vi "backup_EnsTerm.vi"() -> ()   [LabVIEW 2019]
uses:
  <vilib>/Utility/error.llb/DialogType.ctl
  <vilib>/DAQmx/write.llb/DAQmx Write (Digital Bool 1Line 1Point).vi
  <vilib>/DAQmx/write.llb/DAQmx Write (Counter Frequency 1Chan 1Samp).vi
  <vilib>/DAQmx/miscellaneous.llb/DAQmx Fill In Error Info.vi
  <vilib>/DAQmx/create/channels.llb/DAQmx Create Channel (CO-Pulse Generation-Frequency).vi
  <vilib>/DAQmx/configure/timing.llb/DAQmx Timing (Implicit).vi
  <vilib>/addons/control/pid/pid.llb/PID (DBL).vi
  <vilib>/Utility/file.llb/Write Delimited Spreadsheet (string).vi
  <instrlib>/Agilent 34970/Agilent 34970.lvlib
  <resource>/objmgr/daqmx.rc
  <vilib>/addons/control/pid/NI_PID_pid.lvlib
  <instrlib>/Yokogawa WT200 Series/Yokogawa WT200 Series.lvlib
panel:
  out "temperature num cluster":T1
  out "Chart Temperatura":cluster{dbl, dbl, dbl, dbl, dbl, dbl}(graph)={21.505, 22.941, 24.092, 23.94, 23.972, 20.648}
  out "TP 2":dbl
  out "G. TP 2":cluster{dbl, "index":i32}(graph)
  out "TP 15":dbl
  out "TP 13":dbl
  out "TP 12":dbl
  out "TP 11":dbl
  out "TP 10":dbl
  out "TP 8":dbl
  out "TP 7":dbl
  out "TP 6":dbl
  out "TP 5":dbl
  out "TP 3":dbl
  out "TP 1":dbl
  out "G. TP 15":cluster{dbl, "index":i32}(graph)
  out "G. TP 13":cluster{dbl, "index":i32}(graph)
  out "G. TP 12":cluster{dbl, "index":i32}(graph)
  out "G. TP 11":cluster{dbl, "index":i32}(graph)
  out "G. TP 10":cluster{dbl, "index":i32}(graph)
  out "G. TP 8":cluster{dbl, "index":i32}(graph)
  out "G. TP 7":cluster{dbl, "index":i32}(graph)
  out "G. TP 6":cluster{dbl, "index":i32}(graph)
  out "G. TP 5":cluster{dbl, "index":i32}(graph)
  out "G. TP 3":cluster{dbl, "index":i32}(graph)
  out "G. TP 1":cluster{dbl, "index":i32}(graph)
  in  "Idenfier_Ens. Term.":string="medsETMA"
  in  "Idenfier_Freio":string="medsFreio"
  in  "Identifier_Watt":string="medsWatt"
  out "PL(E)":dbl
  out "PC(E)":dbl
  out "PC(T)":dbl
  out "PL(T)":dbl
  out "t":dbl
  out "Tensão de saída":dbl format="%.4f"
  out "Corrente de saída":dbl format="%.4f"
  out "watt num cluster":T2
  in  "Liga Fonte":bool
  out "Resposta":string
  out "Tradução":string
  in  "Parar motor":bool
  in  "Envia mensagem":bool
  in  "Enviar velocidade":bool
  in  "Seta carga":bool
  in  "Limite de tensão":dbl=30.0 min=0.0 max=30.0 step=0.5 format="%.4f"
  in  "Limite de corrente":dbl=0.075 min=0.0 max=0.4 step=0.01 format="%.4f"
  in  "Mensagem":T3(ring)=enum."Read power"
  in  "Velocidade (RPM)":u16=1000 min=1000 max=10000 step=100
  in  "Parâmetros serial":T4={"Serial VCC"="COM7", "timeout"=2, "baud rate"=600, "flow control"=0, "data bits"=8, "parity"=enum."None", "stop bits"=10, "termination char"=FALSE} {"stop bits" items=["1.0"=10, "1.5"=15, "2.0"=20]; "flow control" items=["None", "XON/XOFF", "RTS/CTS", "XON/XOFF & RTS/CTS", "DTR/DSR", "XON/XOFF & DTR/DSR"]}
  in  "Medição contínua? WT230":bool=TRUE
  in  "Realiza medição WT230":bool=TRUE
  out "Chart potencia numeric":T5(graph)={"PC(A)"=0.0, "PC(B)"=7.200000254670158e-05, "PC(T)"=7.200000254670158e-05, "PL(A)"=0.0, "PL(B)"=0.0, "PL(T)"=0.0, "PC(E)"=1.0970638990402222, "PL(E)"=1.0099999904632568}
  out "Chart corrente numeric":cluster{"I(A)":dbl, "I(B)":dbl, "I(E)":dbl}(graph)={"I(A)"=0.0, "I(B)"=0.0, "I(E)"=0.14239999651908875}
  out "Chart tensão numeric":cluster{"V(A)":dbl, "V(B)":dbl, "V(E)":dbl}(graph)={"V(A)"=0.0, "V(B)"=0.0, "V(E)"=228.25999450683594}
  in  "Tempo de integração (s)":u32=5 min=1 max=60 step=1
  in  "SP:":dbl(slide)=25.0 min=0.0 max=0.0 scale=25.0..70.0
  out "MV":dbl(graph)
  in  "Ts":dbl=1.0
  out "PV":dbl
  out "Process variable and Setpoint":cluster{"initial PV":dbl, "SP:":dbl}(graph)
  in  "PID gains":T6={"proportional gain (Kc)"=39.6, "integral time (Ti, min)"=14.617, "derivative time (Td, min)"=0.0} {"derivative time (Td, min)" format="%.3f"; "integral time (Ti, min)" format="%.3f"; "proportional gain (Kc)" format="%.6f"}
  in  "Frequency":dbl=1.0 format="%.6f"
  out "Duty Cycle":sgl=0.1 min=0.1 max=99.9 format="%#_6f"
  in  "Forno_on":bool=TRUE
  out "Iteration":i32
  in  "STOP":bool
  out "Temperature CH4 [degC]":dbl
  out "Temperature CH9 [degC]":dbl
  out "Time":dbl=300.0 format="%<%H:%M:%S>t"
  in  "Idenfier_Forno":string="medsForno"
  # "Temperaturas do Motor/Freio"
  # "Temperaturas dos Termopares"
  # "Gráficos:"
  # "Nome do arquivo:"
  # "Legenda:"
  # "TP 1: Termopar do Capacitor C011"
  # "TP 8: Termopar do CI SMPS IC100"
  # "TP 2: Termopar do Capacitor C009"
  # "TP 10: Termopar do Indutor L100"
  # "TP 3: Termopar do Choke L001"
  # "TP 11: Termopar do Capacitor C112"
  # "TP 5: Termopar do Capacitor C006"
  # "TP 12: Termopar do Capacitor C504"
  # "TP 6: Termopar do Fusível F002"
  # "TP 13: Termopar do Microcontrolador IC601"
  # "TP 7: Termopar do Conector CN204"
  # "TP 15: Termopar do Dissipador"
  # "Freio"
  # "Wattímetro WT230 Yokogawa"
  # "Controle de Temperatura do Forno"
  # "Controles"
  # "Geral"
  # "Respostas do Sistema em Malha Fechada"
  # "Controles"
  # "Medidas"
  # "Respostas temporais"
  # "Medidas"
  # "Controles"
  # "Inversor de Frequência"
  # "Comandos"
  # "Medidas"
  # "Parâmetros Serial"
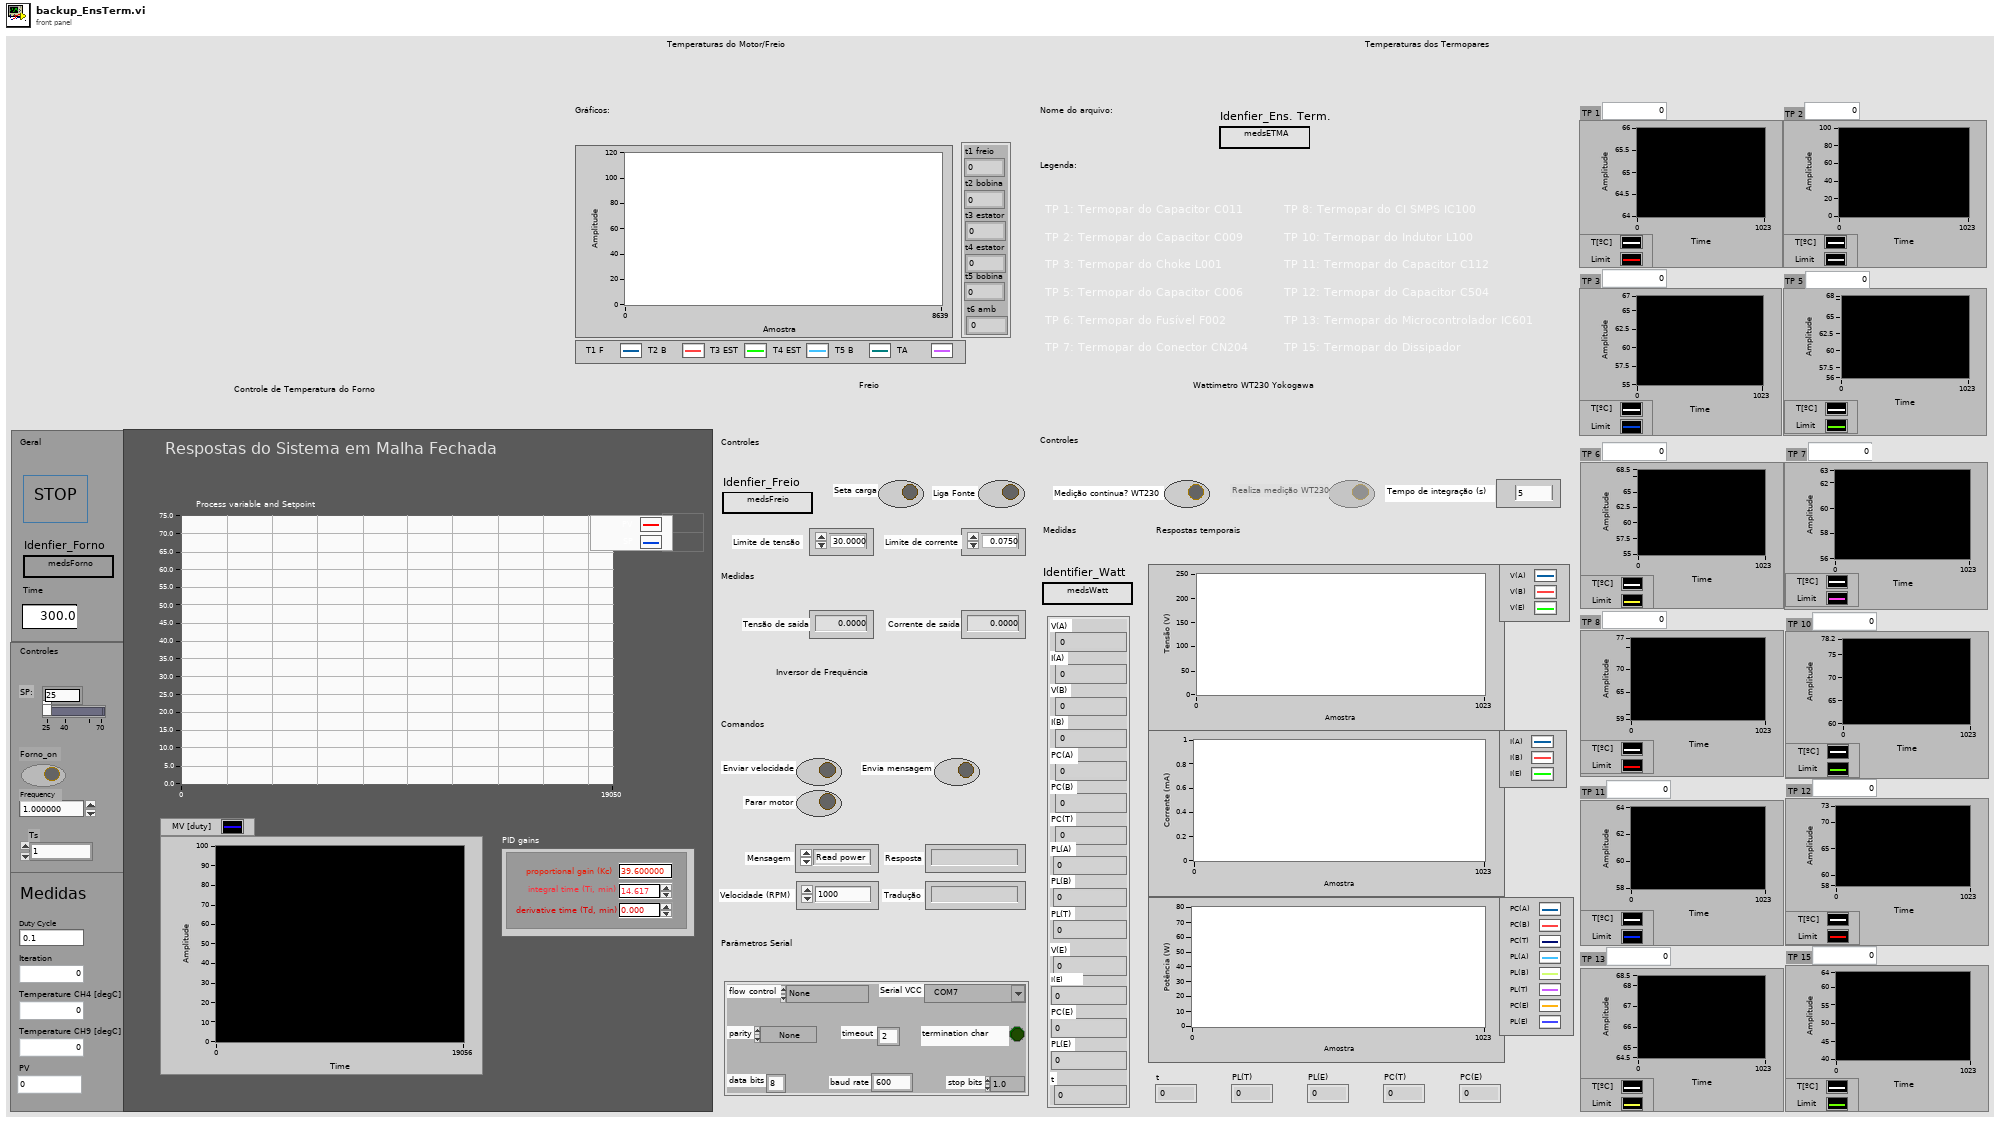
[diagram p1: front panel]
types:
  T1 = cluster{"t1 freio":dbl, "t2 bobina":dbl, "t5 bobina":dbl, "t4 estator":dbl, "t3 estator":dbl, "t6 amb":dbl}
  T2 = cluster{"V(A)":dbl, "I(A)":dbl, "V(B)":dbl, "I(B)":dbl, "PC(A)":dbl, "PC(B)":dbl, "PC(T)":dbl, "PL(T)":dbl, "PL(B)":dbl, "PL(A)":dbl, "V(E)":dbl, "PL(E)":dbl, "PC(E)":dbl, "I(E)":dbl, "t":dbl}
  T3 = enum16{"Read set speed", "Read operation status", "Read power", "Read starting trials", "Read bus voltage", "Read temperature", "Read power limitation", "Read PWM mode", "Read PWM frequency", "Read real speed"}
  T4 = cluster{"Serial VCC":refnum<visa-resource-name>, "timeout":u32, "baud rate":u32, "flow control":u16, "data bits":u16, "parity":enum16{"None", "Odd", "Even", "Mark", "Space"}, "stop bits":u16, "termination char":bool}
  T5 = cluster{"PC(A)":dbl, "PC(B)":dbl, "PC(T)":dbl, "PL(A)":dbl, "PL(B)":dbl, "PL(T)":dbl, "PC(E)":dbl, "PL(E)":dbl}
  T6 = cluster{"proportional gain (Kc)":dbl, "integral time (Ti, min)":dbl, "derivative time (Td, min)":dbl}
  T7 = enum16{"Start Comm.", "End Comm.", "Wait", "Send Static Message", "Set Speed"}
  T8 = enum16{"Thermocouple", "Thermistor", "RTD", "4-Wire RTD", "Default (Last)"}
  T9 = enum8{"Enabled", "Disabled", "Disabled and Grayed Out"}
  T10 = typedef "DialogType.ctl" = u16
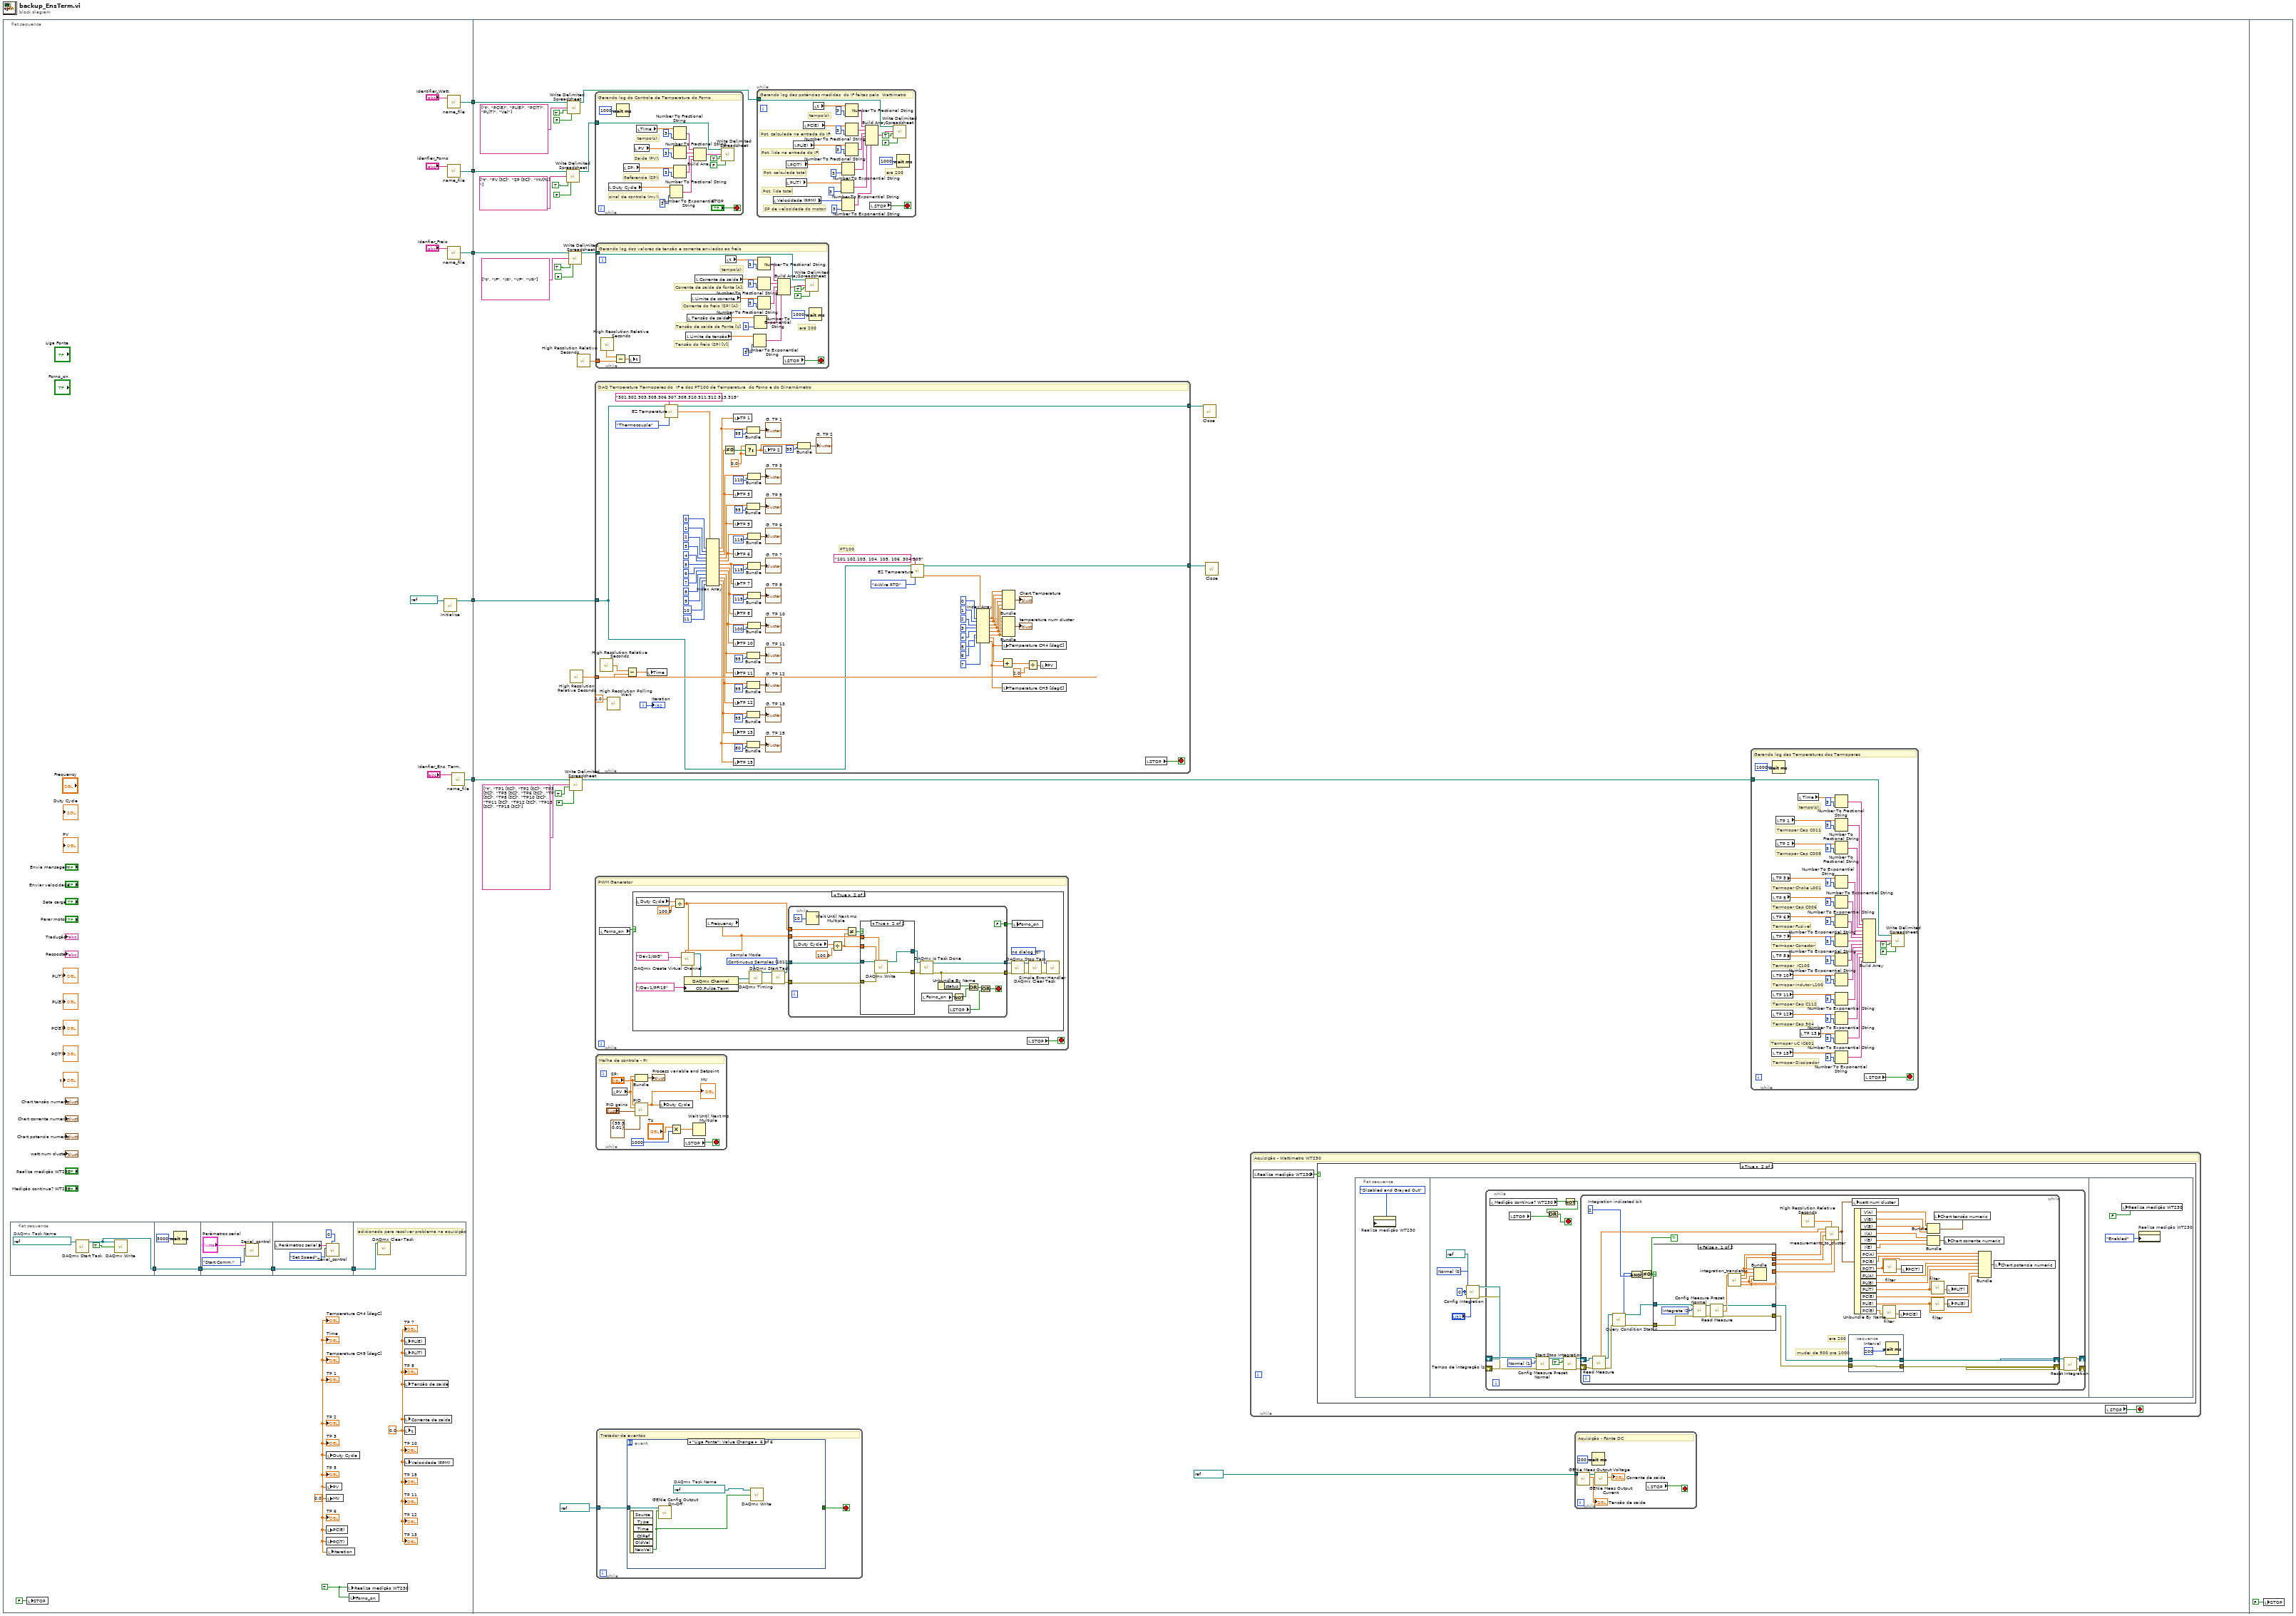
[diagram p0: block diagram]
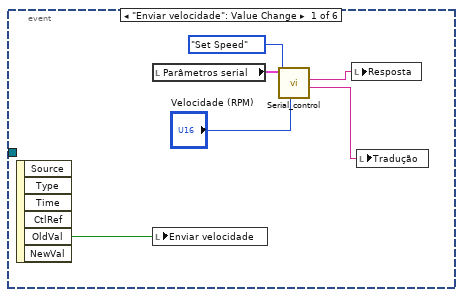
[diagram p2: hidden frame]
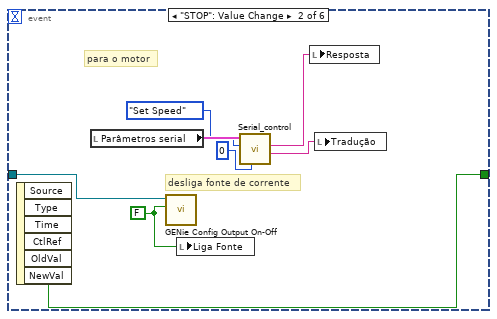
[diagram p3: hidden frame]
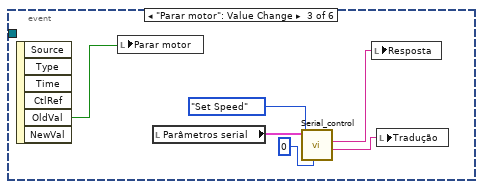
[diagram p4: hidden frame]
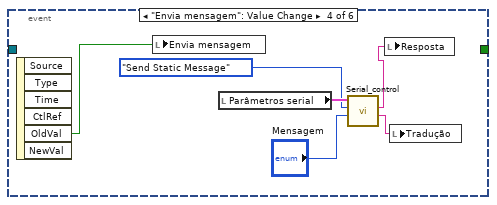
[diagram p5: hidden frame]
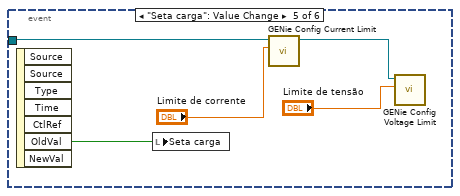
[diagram p6: hidden frame]
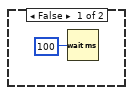
[diagram p7: hidden frame]
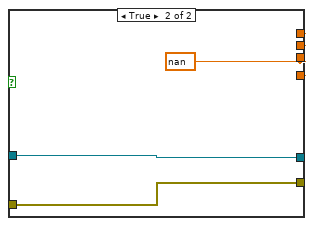
[diagram p8: hidden frame]
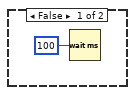
[diagram p9: hidden frame]
diagram:
  n1 = flat-sequence {
    tunnel: [w22] -> w5
    tunnel: [w21] -> w4
    tunnel: [w17] -> w3
    tunnel: [w15] -> w2
    tunnel: [w11] -> w1
    tunnel: w5 -> [w37]
    tunnel: w4 -> [w59]
    tunnel: w3 -> [w56]
    tunnel: w2 -> [w51]
    tunnel: w1 -> [w42]
    frame #0 {
      w13 = 0.0 ("Temperature 1")
      w14 = TRUE ("Realiza medição WT230")
      w10 = 0.0 ("Temperature 1")
      n2 = flat-sequence {
        tunnel: [w24] -> w9
        tunnel: w9 -> [w27]
        tunnel: [w27] -> w8
        tunnel: w8 -> [w29]
        tunnel: [w29] -> w7
        tunnel: w7 -> [w32]
        tunnel: [w32] -> w6
        tunnel: w6 -> [w36]
        frame #0 {
          w25 = refnum<k21> "alimentacao_inversor"  # DAQmx Task Name
          n3 = call <vilib>:"DAQmx Start Task.vi"("task/channels in"=w25) -> ("task out"=w24:refnum<k21>)  [unwired: 13 in, 1 out]
          n4 = call-poly <vilib>:"DAQmx Write.vi"("task/channels in"=w24, "data"=TRUE) -> ()  [unwired: 11 in, 3 out]
        }
        frame #1 {
          n5 = Wait (ms)(milliseconds to wait=u32 3000) -> ()  [unwired: 1 out]
        }
        frame #2 {
          n6 = call "Serial_control.vi"("Função"=T7."Start Comm.", "comm cluster"="Parâmetros serial") -> ()  [unwired: 3 in, 4 out]
        }
        frame #3 {
          n7 = local read "Parâmetros serial"() -> (w34:T4)
          n8 = call "Serial_control.vi"("Enviar número"=u16 0, "Função"=T7."Set Speed", "comm cluster"=w34) -> ()  [unwired: 2 in, 4 out]
        }
        frame #4 {
          # "adicionado para resolver problema na aquisição"
          n9 = call <vilib>:"DAQmx Clear Task.vi"("task in"=w36) -> ()  [unwired: 14 in, 1 out]
        }
      }
      n10 = local write "STOP"(FALSE ("STOP")) -> ()
      n11 = local write "Duty Cycle"(w10) -> ()
      n12 = local write "PV"(w10) -> ()
      n13 = local write "MV"(w10) -> ()
      n14 = local write "PC(E)"(w10) -> ()
      n15 = local write "PC(T)"(w10) -> ()
      n16 = local write "Iteration"(w10) -> ()
      n17 = local write "Realiza medição WT230"(w14) -> ()
      n18 = local write "Forno_on"(w14) -> ()
      n19 = local write "PL(E)"(w13) -> ()
      n20 = local write "PL(T)"(w13) -> ()
      n21 = local write "Tensão de saída"(w13) -> ()
      n22 = local write "Corrente de saída"(w13) -> ()
      n23 = local write "t"(w13) -> ()
      n24 = local write "Velocidade (RPM)"(w13) -> ()
      n25 = call <instrlib>:"Initialize.vi"("VISA Resource Name"=refnum<visa-resource-name> "Agilent" ("VISA AGILENT")) -> ("VISA Resource Name Out"=w22:refnum<visa-resource-name>)  [unwired: 13 in, 1 out]
      n26 = call "name_file.vi"("Identifier"="Identifier_Watt") -> ("appended path"=w17:path)  [unwired: 2 in]
      n27 = call "name_file.vi"("Identifier"="Idenfier_Forno") -> ("appended path"=w21:path)  [unwired: 2 in]
      n28 = call "name_file.vi"("Identifier"="Idenfier_Freio") -> ("appended path"=w15:path)  [unwired: 2 in]
      n29 = call "name_file.vi"("Identifier"="Idenfier_Ens. Term.") -> ("appended path"=w11:path)  [unwired: 2 in]
      "Temperature CH4 [degC]" <- w10
      "Temperature CH9 [degC]" <- w10
      "Time" <- w10
      "TP 1" <- w10
      "TP 2" <- w10
      "TP 3" <- w10
      "TP 5" <- w10
      "TP 6" <- w10
      "TP 7" <- w13
      "TP 8" <- w13
      "TP 10" <- w13
      "TP 11" <- w13
      "TP 12" <- w13
      "TP 13" <- w13
      "TP 15" <- w13
    }
    frame #1 {
      n30 = call-poly <vilib>:"Write Delimited Spreadsheet.vi"("file path (dialog if empty)"=w59, "1D data"=string[] ["t", "PV [ºC]", "SP [ºC]", "MV[%] "] ("appended array"), "append to file? (new file:F)"=TRUE, "transpose? (no:F)"=FALSE) -> ("new file path (Not A Path if cancelled)"=w60:path)  [unwired: 10 in, 1 out]
      n31 = call-poly <vilib>:"Write Delimited Spreadsheet.vi"("file path (dialog if empty)"=w56, "1D data"=string[] ["t", "PC(E)", "PL(E)", "PC(T)", "PL(T)", "Vel"] ("appended array"), "append to file? (new file:F)"=TRUE, "transpose? (no:F)"=FALSE) -> ("new file path (Not A Path if cancelled)"=w52:path)  [unwired: 10 in, 1 out]
      n32 = call-poly <vilib>:"Write Delimited Spreadsheet.vi"("file path (dialog if empty)"=w51, "1D data"=string[] ["t", "IF", "IR", "VF", "VR"] ("appended array"), "append to file? (new file:F)"=TRUE, "transpose? (no:F)"=FALSE) -> ("new file path (Not A Path if cancelled)"=w47:path)  [unwired: 10 in, 1 out]
      n33 = call-poly <vilib>:"Write Delimited Spreadsheet.vi"("file path (dialog if empty)"=w42, "1D data"=string[] ["t", "TP1 [ºC]", "TP2 [ºC]", "TP3 [ºC]", "TP5 [ºC]", "TP6 [ºC]", "TP7 [ºC]", "TP8 [ºC]", "TP10 [ºC]", "TP11 [ºC]", "TP12 [ºC]", "TP13 [ºC]", "TP15 [ºC]"] ("appended array"), "append to file? (new file:F)"=TRUE, "transpose? (no:F)"=FALSE) -> ("new file path (Not A Path if cancelled)"=w41:path)  [unwired: 10 in, 1 out]
      n34 = call <vilib>:"High Resolution Relative Seconds.vi"() -> ("relative seconds"=w39:dbl)
      n35 = call <vilib>:"High Resolution Relative Seconds.vi"() -> ("relative seconds"=w46:dbl)
      n36 = while {
        tunnel: w60 -> [w453]
        stop <- "STOP" stop-if-true
        # "tempo(s):"
        # "Saída (PV):"
        # "Referencia (SP):"
        # "sinal de controle (mv):"
        # "Gerando log do Controle de Temperatura do Forno"
        n37 = local read "Duty Cycle"() -> (w449:sgl)
        n38 = Wait (ms)(milliseconds to wait=u32 1000) -> ()  [unwired: 1 out]
        n39 = local read "SP:"() -> (w442:dbl)
        n40 = local read "PV"() -> (w448:dbl)
        n41 = local read "Time"() -> (w446:dbl)
        n42 = Number To Exponential String(number=w449, precision (6)=i16 3) -> (E-format string=w451:string)  [unwired: 2 in]
        n43 = Number To Fractional String(number=w446, precision (6)=i16 3) -> (F-format string=w445:string)  [unwired: 2 in]
        n44 = Number To Fractional String(number=w448, precision (6)=i16 3) -> (F-format string=w444:string)  [unwired: 2 in]
        n45 = Number To Fractional String(number=w442, precision (6)=i16 3) -> (F-format string=w440:string)  [unwired: 2 in]
        n46 = Build Array(w445, w444, w440, w451) -> (w441:string[])
        n47 = call-poly <vilib>:"Write Delimited Spreadsheet.vi"("file path (dialog if empty)"=w453, "1D data"=w441, "append to file? (new file:F)"=TRUE, "transpose? (no:F)"=FALSE) -> ()  [unwired: 10 in, 2 out]
      }
      n48 = while {
        tunnel: [w133] -> w40
        tunnel: w39 -> [w67]
        tunnel: [w66] -> w38
        tunnel: w37 -> [w64]
        i -> [w65]
        stop <- w136 stop-if-true
        w130 = 0.0 ("t")
        # "PT100"
        # "DAQ Temperatura Termopares do  IF e dos PT100 de Temperatura  do Forno e do Dinamômetro"
        n49 = call <vilib>:"High Resolution Relative Seconds.vi"() -> ("relative seconds"=w83:dbl)
        n50 = call <vilib>:"High Resolution Polling Wait.vi"("seconds to wait"=1.0) -> ()  [unwired: 10 in, 1 out]
        n51 = Subtract(x=w83, y=w67) -> (x-y=w79:dbl)
        n52 = local write "Time"(w79) -> ()
        n53 = call <instrlib>:"EZ Temperature.vi"("VISA Resource Name"=w64, "Scan List (empty)"="301,302,303,305,306,307,308,310,311,312,313,315", "Transducer Type (4:Def-Last)"=T8."Thermocouple") -> ("VISA Resource Name Out"=w133:refnum<visa-resource-name>, "Output Array"=w139:dbl[])  [unwired: 10 in, 1 out]
        n54 = Index Array(array=w139, index #1=0 ("index"), index #2=1 ("index"), index #3=2 ("index"), index #4=3 ("index"), index #5=4 ("index"), index #6=5 ("index"), index #7=6 ("index"), index #8=7 ("index"), index #9=8 ("index"), index #10=9 ("index"), index #11=10 ("index"), index #12=11 ("index")) -> (element #1=w129:dbl, element #2=w132:dbl, element #3=w106:dbl, element #4=w105:dbl, element #5=w104:dbl, element #6=w103:dbl, element #7=w102:dbl, element #8=w101:dbl, element #9=w100:dbl, element #10=w99:dbl, element #11=w98:dbl, element #12=w97:dbl)
        n55 = Not Equal To 0?(x=w132) -> (x != 0?=w131:bool)
        n56 = local write "TP 1"(w129) -> ()
        n57 = local write "TP 3"(w106) -> ()
        n58 = local write "TP 5"(w105) -> ()
        n59 = local write "TP 6"(w104) -> ()
        n60 = local write "TP 7"(w103) -> ()
        n61 = local write "TP 8"(w102) -> ()
        n62 = local write "TP 10"(w101) -> ()
        n63 = local write "TP 11"(w100) -> ()
        n64 = local write "TP 12"(w99) -> ()
        n65 = local write "TP 13"(w98) -> ()
        n66 = local write "TP 15"(w97) -> ()
        n67 = Select(t=w130, s=w131, f=w130) -> (s? t:f=w96:dbl)
        n68 = Bundle(w129, "index"=95) -> (→"G. TP 1":cluster{dbl, "index":i32})  [unwired: 1 in]
        n69 = Bundle(w105, "index"=95) -> (→"G. TP 5":cluster{dbl, "index":i32})  [unwired: 1 in]
        n70 = Bundle(w100, "index"=95) -> (→"G. TP 11":cluster{dbl, "index":i32})  [unwired: 1 in]
        n71 = Bundle(w99, "index"=95) -> (→"G. TP 12":cluster{dbl, "index":i32})  [unwired: 1 in]
        n72 = Bundle(w98, "index"=95) -> (→"G. TP 13":cluster{dbl, "index":i32})  [unwired: 1 in]
        n73 = Bundle(w97, "index"=80) -> (→"G. TP 15":cluster{dbl, "index":i32})  [unwired: 1 in]
        n74 = Bundle(w106, "index"=110) -> (→"G. TP 3":cluster{dbl, "index":i32})  [unwired: 1 in]
        n75 = Bundle(w104, "index"=115) -> (→"G. TP 6":cluster{dbl, "index":i32})  [unwired: 1 in]
        n76 = Bundle(w103, "index"=115) -> (→"G. TP 7":cluster{dbl, "index":i32})  [unwired: 1 in]
        n77 = Bundle(w102, "index"=115) -> (→"G. TP 8":cluster{dbl, "index":i32})  [unwired: 1 in]
        n78 = Bundle(w101, "index"=100) -> (→"G. TP 10":cluster{dbl, "index":i32})  [unwired: 1 in]
        n79 = local write "TP 2"(w96) -> ()
        n80 = Bundle("t"=w96, "index"=95) -> (→"G. TP 2":cluster{"t":dbl, "index":i32})  [unwired: 1 in]
        n81 = call <instrlib>:"EZ Temperature.vi"("VISA Resource Name"=w64, "Scan List (empty)"="101,102,103, 104, 105, 106, 304,309", "Transducer Type (4:Def-Last)"=T8."4-Wire RTD") -> ("VISA Resource Name Out"=w66:refnum<visa-resource-name>, "Output Array"=w80:dbl[])  [unwired: 10 in, 1 out]
        n82 = Index Array(array=w80, index #1=0 ("index"), index #2=1 ("index"), index #3=2 ("index"), index #4=3 ("index"), index #5=4 ("index"), index #6=5 ("index"), index #7=6 ("index"), index #8=7 ("index")) -> (element #1=w86:dbl, element #2=w87:dbl, element #3=w88:dbl, element #4=w89:dbl, element #5=w90:dbl, element #6=w91:dbl, element #7=w92:dbl, element #8=w93:dbl)
        n83 = Add(x=w92, y=w93) -> (x+y=w81:dbl)
        n84 = Bundle(w86, w87, w88, w89, w90, w91) -> (→"Chart Temperatura":cluster{dbl, dbl, dbl, dbl, dbl, dbl})  [unwired: 1 in]
        n85 = Bundle(w86, w87, w88, w89, w90, w91) -> (→"temperature num cluster":cluster{dbl, dbl, dbl, dbl, dbl, dbl})  [unwired: 1 in]
        n86 = local write "Temperature CH4 [degC]"(w92) -> ()
        n87 = local write "Temperature CH9 [degC]"(w93) -> ()
        n88 = Divide(x=w81, y=2.0) -> (x/y=w82:dbl)
        n89 = local write "PV"(w82) -> ()
        n90 = local read "STOP"() -> (w136:bool)
        "Iteration" <- w65
      }
      n91 = while {
        stop <- w385 stop-if-true
        # "PWM Generator"
        n92 = local read "Forno_on"() -> (w386:bool)
        n93 = case shown="True" w386 {
          frame False {
            n94 = Wait (ms)(milliseconds to wait=u32 100) -> ()  [unwired: 1 out]
          }
          frame True {
            w394 = T10 0 items=["no dialog", "OK message", "continue or stop message", "OK message + warnings", "continue/stop + warnings"] ("type of dialog (OK msg:1)")
            w405 = 10123 items=["Finite Samples"=10178, "Continuous Samples"=10123, "Hardware Timed Single Point"=12522]  # Sample Mode
            n95 = local read "Duty Cycle"() -> (w389:sgl)
            n96 = Divide(x=w389, y=100.0) -> (x/y=w388:dbl)
            n97 = local read "Frequency"() -> (w391:dbl)
            n98 = call-poly <vilib>:"DAQmx Create Virtual Channel.vi"("frequency"=w391, "duty cycle"=w388, "counter"=tag "Dev1/ctr3" ("Counter")) -> ("task out"=w408:refnum<k21>, "error out"=w407:errorcluster)  [unwired: 11 in]
            n99 = property class="DAQmx Channel"(reference=w408, error in=w407, "CO.Pulse.Term"=tag "/Dev1/PFI15" ("Output Terminal")) -> (reference out=w404:refnum<k21>, error out=w403:errorcluster)
            n100 = call-poly <vilib>:"DAQmx Timing.vi"("task/channels in"=w404, "sample mode"=w405, "error in"=w403) -> ("task out"=w402:refnum<k21>, "error out"=w401:errorcluster)  [unwired: 11 in]
            n101 = call <vilib>:"DAQmx Start Task.vi"("task/channels in"=w402, "error in"=w401) -> ("task out"=w400:refnum<k21>, "error out"=w399:errorcluster)  [unwired: 12 in]
            n102 = while {
              tunnel: w400 -> [w419]
              tunnel: w399 -> [w417]
              tunnel: [w428] -> w396
              tunnel: [w429] -> w397
              tunnel: [FALSE ("Liga aquecedor")] -> w393
              tunnel: w388 -> [w415]
              tunnel: w391 -> [w413]
              stop <- w422 stop-if-true
              n103 = local read "Duty Cycle"() -> (w412:sgl)
              n104 = Wait Until Next ms Multiple(millisecond multiple=u32 10) -> ()  [unwired: 1 out]
              n105 = Divide(x=w412, y=100.0) -> (x/y=w410:dbl)
              n106 = Not Equal?(x=w415, y=w410) -> (x != y?=w414:bool)
              n107 = case shown="True" w414 {
                tunnel: [w431 w434] -> w418
                tunnel: w419 -> [w431 w435]
                tunnel: [w430 w436] -> w416
                tunnel: w417 -> [w430 w437]
                tunnel: w410 -> [_ w433]
                tunnel: w413 -> [_ w432]
                frame False {
                }
                frame True {
                  n108 = call-poly <vilib>:"DAQmx Write.vi"("task/channels in"=w435, "frequency"=w432, "duty cycle"=w433, "error in"=w437) -> ("task out"=w434:refnum<k21>, "error out"=w436:errorcluster)  [unwired: 9 in, 1 out]
                }
              }
              n109 = call <vilib>:"DAQmx Is Task Done.vi"("task/channels in"=w418, "error in"=w416) -> ("task out"=w429:refnum<k21>, "error out"=w428:errorcluster)  [unwired: 11 in, 1 out]
              n110 = local read "Forno_on"() -> (w425:bool)
              n111 = Unbundle By Name(w428) -> ("status"=w427:bool)
              n112 = local read "STOP"() -> (w420:bool)
              n113 = Not(x=w425) -> (.not. x?=w423:bool)
              n114 = Or(x=w427, y=w423) -> (x .or. y?=w421:bool)
              n115 = Or(x=w421, y=w420) -> (x .or. y?=w422:bool)
            }
            n116 = call <vilib>:"DAQmx Stop Task.vi"("task/channels in"=w397, "error in"=w396) -> ("task out"=w392:refnum<k21>, "error out"=w398:errorcluster)  [unwired: 12 in]
            n117 = local write "Forno_on"(w393) -> ()
            n118 = call <vilib>:"DAQmx Clear Task.vi"("task in"=w392, "error in"=w398) -> ("error out"=w395:errorcluster)  [unwired: 13 in]
            n119 = call <vilib>:"Simple Error Handler.vi"("error code (no error:0)"=w394, "error in (no error)"=w395) -> ()  [unwired: 3 in, 5 out]
          }
        }
        n120 = local read "STOP"() -> (w385:bool)
      }
      n121 = while {
        stop <- w377 stop-if-true
        # "Malha de controle - PI"
        n122 = local read "PV"() -> (w381:dbl)
        n123 = Bundle("PV"=w381, "SP:"="SP:") -> (→"Process variable and Setpoint":cluster{"PV":dbl, "SP:":dbl})  [unwired: 1 in]
        n124 = call-poly <vilib>:"PID.vi"("output range"=cluster{"output high":dbl, "output low":dbl} {"output high"=99.9, "output low"=0.01}, "PID gains"="PID gains", "process variable"=w381, "setpoint"="SP:") -> ("output"=w376:dbl)  [unwired: 6 in, 1 out]
        "MV" <- w376
        n125 = local write "Duty Cycle"(w376) -> ()
        n126 = Multiply(x="Ts", y=u32 1000 ("unsigned 32bit integer")) -> (x*y=w375:dbl)
        n127 = local read "STOP"() -> (w377:bool)
        n128 = Wait Until Next ms Multiple(millisecond multiple=w375) -> ()  [unwired: 1 out]
      }
      n129 = while {
        tunnel: w47 -> [w217]
        tunnel: w46 -> [w197]
        stop <- w203 stop-if-true
        # "era 200"
        # "Tensão do freio (SP) [V]:"
        # "tempo(s):"
        # "Corrente de saída da fonte [A]:"
        # "Corrente do freio (SP) [A]:"
        # "Tensão de saída da Fonte [V]"
        # "Gerando log dos valores de tensão e corrente enviados ao freio"
        n130 = call <vilib>:"High Resolution Relative Seconds.vi"() -> ("relative seconds"=w198:dbl)
        n131 = Subtract(x=w198, y=w197) -> (x-y=w196:dbl)
        n132 = local write "t"(w196) -> ()
        n133 = local read "Limite de tensão"() -> (w201:dbl)
        n134 = local read "Tensão de saída"() -> (w213:dbl)
        n135 = local read "Limite de corrente"() -> (w206:dbl)
        n136 = local read "Corrente de saída"() -> (w212:dbl)
        n137 = local read "t"() -> (w210:dbl)
        n138 = Number To Exponential String(number=w201, precision (6)=i16 3) -> (E-format string=w199:string)  [unwired: 2 in]
        n139 = Number To Exponential String(number=w213, precision (6)=i16 3) -> (E-format string=w215:string)  [unwired: 2 in]
        n140 = Number To Fractional String(number=w210, precision (6)=i16 3) -> (F-format string=w209:string)  [unwired: 2 in]
        n141 = Number To Fractional String(number=w212, precision (6)=i16 3) -> (F-format string=w208:string)  [unwired: 2 in]
        n142 = Number To Fractional String(number=w206, precision (6)=i16 3) -> (F-format string=w204:string)  [unwired: 2 in]
        n143 = Build Array(w209, w208, w204, w215, w199) -> (w205:string[])
        n144 = local read "STOP"() -> (w203:bool)
        n145 = call-poly <vilib>:"Write Delimited Spreadsheet.vi"("file path (dialog if empty)"=w217, "1D data"=w205, "append to file? (new file:F)"=TRUE, "transpose? (no:F)"=FALSE) -> ()  [unwired: 10 in, 2 out]
        n146 = Wait (ms)(milliseconds to wait=u32 1000) -> ()  [unwired: 1 out]
      }
      n147 = while {
        tunnel: refnum<visa-resource-name> "Lambda" ("VISA name") -> [w250]
        stop <- w251 stop-if-true
        # "Tratador de eventos"
        n148 = event shown="[5] \"Liga Fonte\": Value Change" {
          selector: _ -> [_ _ _ _ _ _]
          dyn-events: _ -> [_ _ _ _ _ _]
          timeout: _ -> [_ _ _ _ _ _]
          tunnel: w250 -> [_ w259 _ _ w279 w285]
          tunnel: [_ w260 _ _ _ _] -> w251
          event "Enviar velocidade": Value Change {
            n149 = event-data() -> ("OldVal"=w257:bool)  [unwired: 1 in, 5 out]
            n150 = local read "Parâmetros serial"() -> (w256:T4)
            n151 = local write "Enviar velocidade"(w257) -> ()
            n152 = call "Serial_control.vi"("Enviar número"="Velocidade (RPM)", "Função"=T7."Set Speed", "comm cluster"=w256) -> ("translated message"=w253:string, "read buffer"=w254:string)  [unwired: 2 in, 2 out]
            n153 = local write "Resposta"(w254) -> ()
            n154 = local write "Tradução"(w253) -> ()
          }
          event "STOP": Value Change {
            w258 = FALSE ("Output ON")
            # "desliga fonte de corrente"
            # "para o motor"
            n155 = event-data() -> ("NewVal"=w260:bool)  [unwired: 1 in, 5 out]
            n156 = local read "Parâmetros serial"() -> (w265:T4)
            n157 = call <instrlib>:"GENie Config Output On-Off.vi"("Output ON"=w258, "VISA"=w259) -> ()  [unwired: 8 in, 2 out]
            n158 = local write "Liga Fonte"(w258) -> ()
            n159 = call "Serial_control.vi"("Enviar número"=u16 0, "Função"=T7."Set Speed", "comm cluster"=w265) -> ("translated message"=w263:string, "read buffer"=w264:string)  [unwired: 2 in, 2 out]
            n160 = local write "Resposta"(w264) -> ()
            n161 = local write "Tradução"(w263) -> ()
          }
          event "Parar motor": Value Change {
            n162 = event-data() -> ("OldVal"=w268:bool)  [unwired: 1 in, 5 out]
            n163 = local write "Parar motor"(w268) -> ()
            n164 = local read "Parâmetros serial"() -> (w271:T4)
            n165 = call "Serial_control.vi"("Enviar número"=u16 0, "Função"=T7."Set Speed", "comm cluster"=w271) -> ("translated message"=w266:string, "read buffer"=w267:string)  [unwired: 2 in, 2 out]
            n166 = local write "Resposta"(w267) -> ()
            n167 = local write "Tradução"(w266) -> ()
          }
          event "Envia mensagem": Value Change {
            n168 = event-data() -> ("OldVal"=w277:bool)  [unwired: 1 in, 5 out]
            n169 = local write "Envia mensagem"(w277) -> ()
            n170 = local read "Parâmetros serial"() -> (w276:T4)
            n171 = call "Serial_control.vi"("Message"="Mensagem", "Função"=T7."Send Static Message", "comm cluster"=w276) -> ("translated message"=w274:string, "read buffer"=w273:string)  [unwired: 2 in, 2 out]
            n172 = local write "Resposta"(w273) -> ()
            n173 = local write "Tradução"(w274) -> ()
          }
          event "Seta carga": Value Change {
            n174 = event-data() -> ("OldVal"=w280:bool)  [unwired: 1 in, 6 out]
            n175 = local write "Seta carga"(w280) -> ()
            n176 = call <instrlib>:"GENie Config Current Limit.vi"("Current Limit"="Limite de corrente", "VISA"=w279) -> ("VISA out"=w278:refnum<visa-resource-name>)  [unwired: 8 in, 1 out]
            n177 = call <instrlib>:"GENie Config Voltage Limit.vi"("Volt Limit"="Limite de tensão", "VISA"=w278) -> ()  [unwired: 8 in, 2 out]
          }
          event "Liga Fonte": Value Change {
            w284 = refnum<k21> "resfriamento_freio"  # DAQmx Task Name
            n178 = event-data() -> ("NewVal"=w283:bool)  [unwired: 1 in, 5 out]
            n179 = call <instrlib>:"GENie Config Output On-Off.vi"("Output ON"=w283, "VISA"=w285) -> ()  [unwired: 8 in, 2 out]
            n180 = call-poly <vilib>:"DAQmx Write.vi"("task/channels in"=w284, "data"=w283) -> ()  [unwired: 11 in, 3 out]
          }
        }
      }
      n181 = while {
        tunnel: w52 -> [w241]
        stop <- w227 stop-if-true
        # "era 200"
        # "SP de velocidade do motor:"
        # "Pot. lida total"
        # "tempo(s):"
        # "Pot. calculada na entrada do IF:"
        # "Pot. lida na entrada do IF:"
        # "Pot. calculada total"
        # "Gerando log das potências medidas  do IF feitas pelo  Wattímetro"
        n182 = local read "Velocidade (RPM)"() -> (w223:u16)
        n183 = local read "PL(T)"() -> (w226:dbl)
        n184 = local read "PC(T)"() -> (w237:dbl)
        n185 = local read "PL(E)"() -> (w230:dbl)
        n186 = local read "PC(E)"() -> (w236:dbl)
        n187 = local read "t"() -> (w234:dbl)
        n188 = Number To Exponential String(number=w226, precision (6)=i16 3) -> (E-format string=w224:string)  [unwired: 2 in]
        n189 = Number To Exponential String(number=w237, precision (6)=i16 3) -> (E-format string=w239:string)  [unwired: 2 in]
        n190 = Number To Exponential String(number=w223, precision (6)=i16 3) -> (E-format string=w220:string)  [unwired: 2 in]
        n191 = Number To Fractional String(number=w234, precision (6)=i16 3) -> (F-format string=w233:string)  [unwired: 2 in]
        n192 = Number To Fractional String(number=w236, precision (6)=i16 3) -> (F-format string=w232:string)  [unwired: 2 in]
        n193 = Number To Fractional String(number=w230, precision (6)=i16 3) -> (F-format string=w228:string)  [unwired: 2 in]
        n194 = Build Array(w233, w232, w228, w239, w224, w220) -> (w229:string[])
        n195 = local read "STOP"() -> (w227:bool)
        n196 = call-poly <vilib>:"Write Delimited Spreadsheet.vi"("file path (dialog if empty)"=w241, "1D data"=w229, "append to file? (new file:F)"=TRUE, "transpose? (no:F)"=FALSE) -> ()  [unwired: 10 in, 2 out]
        n197 = Wait (ms)(milliseconds to wait=u32 1000) -> ()  [unwired: 1 out]
      }
      n198 = call <instrlib>:"Close.vi"("VISA Resource Name"=w40) -> ()  [unwired: 14 in, 1 out]
      n199 = call <instrlib>:"Close.vi"("VISA Resource Name"=w38) -> ()  [unwired: 14 in, 1 out]
      n200 = while {
        stop <- w286 stop-if-true
        # "Aquisição - Wattímetro WT230"
        n201 = local read "Realiza medição WT230"() -> (w287:bool)
        n202 = case shown="True" w287 {
          frame False {
            n203 = Wait (ms)(milliseconds to wait=u32 100) -> ()  [unwired: 1 out]
          }
          frame True {
            n204 = flat-sequence {
              frame #0 {
                n205 = property on="Realiza medição WT230" class="Bool (strict)"("DisabledEnum"=T9."Disabled and Grayed Out" ("Disabled")) -> ()  [unwired: 2 in, 2 out]
              }
              frame #1 {
                w292 = u16 0 items=["Normal", "Continuous"] ("Integ Mode (0: Normal)")
                w293 = u32 0 ("Hour (0)")
                n206 = call <instrlib>:"Config Integration.vi"("VISA resource name"=refnum<visa-resource-name> "WT", "Integ Mode (0: Normal)"=w292, "Hour (0)"=w293, "Minute (0)"=w293, "Second (0)"="Tempo de integração (s)") -> ("VISA resource name out"=w295:refnum<visa-resource-name>, "error out"=w294:errorcluster)  [unwired: 9 in]
                n207 = while {
                  shift-right: [w299] -> _
                  shift-left: w295 -> [w297]
                  shift-right: [w298] -> _
                  shift-left: w294 -> [w296]
                  stop <- w300 stop-if-true
                  w306 = u16 1 items=["Clear", "Normal", "Integrate"] ("Preset Pattern (0: Clear)")
                  n208 = local read "Medição contínua? WT230"() -> (w302:bool)
                  n209 = local read "STOP"() -> (w303:bool)
                  n210 = call <instrlib>:"Config Measure Preset Normal.vi"("VISA resource name"=w297, "Preset Pattern (0: Clear)"=w306, "error in (no error)"=w296) -> ("VISA resource name out"=w308:refnum<visa-resource-name>, "error out"=w307:errorcluster)  [unwired: 11 in]
                  n211 = call <instrlib>:"Start Stop Integration.vi"("VISA resource name"=w308, "Start/Stop (F: Stop)"=TRUE, "error in (no error)"=w307) -> ("VISA resource name out"=w311:refnum<visa-resource-name>, "error out"=w310:errorcluster)  [unwired: 11 in]
                  n212 = Not(x=w302) -> (.not. x?=w301:bool)
                  n213 = Or(x=w301, y=w303) -> (x .or. y?=w300:bool)
                  n214 = while {
                    shift-left: w311 -> [w351]
                    shift-right: [w339] -> w305
                    shift-left: w310 -> [w348]
                    shift-right: [w337] -> w304
                    stop <- w347 continue-if-true
                    w354 = u16 2  # Integration indicated bit
                    # "era 200"
                    # "mudei de 500 pra 1000"
                    n215 = call <instrlib>:"Read Measure.vi"("VISA resource name"=w351, "error in (no error)"=w348) -> ("VISA resource name out"=w350:refnum<visa-resource-name>, "Measure Value"=w341:sgl[], "error out"=w349:errorcluster)  [unwired: 10 in, 1 out]
                    n216 = call <instrlib>:"Query Condition Status.vi"("VISA resource name"=w350, "error in (no error)"=w349) -> ("VISA resource name out"=w336:refnum<visa-resource-name>, "Condition"=w352:u16, "error out"=w335:errorcluster)  [unwired: 11 in]
                    n217 = And(x=w352, y=w354) -> (x .and. y?=w353:u16)
                    n218 = Not Equal To 0?(x=w353) -> (x != 0?=w347:bool)
                    n219 = case shown="False" w347 {
                      tunnel: [w365 w372] -> w346
                      tunnel: [w364 w372] -> w345
                      tunnel: [w363 w372] -> w344
                      tunnel: [w362 w372] -> w343
                      tunnel: [w361 w371] -> w340
                      tunnel: [w360 w370] -> w338
                      tunnel: w336 -> [w359 w371]
                      tunnel: w335 -> [w358 w370]
                      frame False {
                        w366 = u16 2 items=["Clear", "Normal", "Integrate"] ("Preset Pattern (0: Clear)")
                        n220 = call <instrlib>:"Config Measure Preset Normal.vi"("VISA resource name"=w359, "Preset Pattern (0: Clear)"=w366, "error in (no error)"=w358) -> ("VISA resource name out"=w369:refnum<visa-resource-name>, "error out"=w368:errorcluster)  [unwired: 11 in]
                        n221 = call <instrlib>:"Read Measure.vi"("VISA resource name"=w369, "error in (no error)"=w368) -> ("VISA resource name out"=w361:refnum<visa-resource-name>, "Measure Value"=w367:sgl[], "error out"=w360:errorcluster)  [unwired: 10 in, 1 out]
                        n222 = call "integration_translator.vi"("Valores integração"=w367) -> ("PI(E)"=w362:sgl, "PI(T)"=w363:sgl, "PI(B)"=w364:sgl, "PI(A)"=w365:sgl)  [unwired: 7 in]
                        n223 = Bundle("PI(A)"=w365, "PI(B)"=w364, "PI(T)"=w363, "PI(E)"=w362) -> ()  [unwired: 1 in, 1 out]
                      }
                      frame True {
                        w372 = nan
                      }
                    }
                    n224 = call <vilib>:"High Resolution Relative Seconds.vi"() -> ("relative seconds"=w342:dbl)
                    n225 = call "measurements_to_cluster.vi"("PI(E)"=w343, "PI(T)"=w344, "relative seconds"=w342, "PI(B)"=w345, "PI(A)"=w346, "Measure Value"=w341) -> ("watt cluster"=w334:T2)  [unwired: 4 in, 1 out]
                    n226 = stacked-sequence {
                      tunnel: w340 -> [w356]
                      tunnel: [w356] -> w339
                      tunnel: w338 -> [w355]
                      tunnel: [w355] -> w337
                      frame #0 {
                        w357 = u32 200  # Interval
                        n227 = Wait (ms)(milliseconds to wait=w357) -> ()  [unwired: 1 out]
                      }
                    }
                    n228 = local write "watt num cluster"(w334) -> ()
                    n229 = Unbundle By Name(w334) -> ("V(A)"=w329:dbl, "V(B)"=w328:dbl, "V(E)"=w327:dbl, "I(A)"=w326:dbl, "I(B)"=w325:dbl, "I(E)"=w324:dbl, "PC(A)"=w323:dbl, "PC(B)"=w322:dbl, "PC(T)"=w321:dbl, "PL(A)"=w319:dbl, "PL(B)"=w318:dbl, "PL(T)"=w317:dbl, "PC(E)"=w316:dbl, "PL(E)"=w315:dbl, "PC(E)"=w313:dbl)
                    n230 = call "filter.vi"("input"=w313) -> ("output"=w312:dbl)  [unwired: 10 in]
                    n231 = call "filter.vi"("input"=w321) -> ("output"=w320:dbl)  [unwired: 10 in]
                    n232 = local write "PC(E)"(w312) -> ()
                    n233 = local write "PC(T)"(w320) -> ()
                    n234 = Bundle("V(A)"=w329, "V(B)"=w328, "V(E)"=w327) -> (w333:cluster{"V(A)":dbl, "V(B)":dbl, "V(E)":dbl})  [unwired: 1 in]
                    n235 = Bundle("I(A)"=w326, "I(B)"=w325, "I(E)"=w324) -> (w332:cluster{"I(A)":dbl, "I(B)":dbl, "I(E)":dbl})  [unwired: 1 in]
                    n236 = call "filter.vi"("input"=w317) -> ("output"=w331:dbl)  [unwired: 10 in]
                    n237 = call "filter.vi"("input"=w315) -> ("output"=w330:dbl)  [unwired: 10 in]
                    n238 = local write "Chart tensão numeric"(w333) -> ()
                    n239 = local write "Chart corrente numeric"(w332) -> ()
                    n240 = local write "PL(T)"(w331) -> ()
                    n241 = local write "PL(E)"(w330) -> ()
                    n242 = Bundle("PC(A)"=w323, "PC(B)"=w322, "PC(T)"=w321, "PL(A)"=w319, "PL(B)"=w318, "PL(T)"=w317, "PC(E)"=w316, "PL(E)"=w315) -> (w314:T5)  [unwired: 1 in]
                    n243 = local write "Chart potencia numeric"(w314) -> ()
                  }
                  n244 = call <instrlib>:"Reset Integration.vi"("VISA resource name"=w305, "error in (no error)"=w304) -> ("VISA resource name out"=w299:refnum<visa-resource-name>, "error out"=w298:errorcluster)  [unwired: 12 in]
                }
              }
              frame #2 {
                n245 = local write "Realiza medição WT230"(FALSE ("Realiza medição")) -> ()
                n246 = property on="Realiza medição WT230" class="Bool (strict)"("DisabledEnum"=T9."Enabled" ("Disabled")) -> ()  [unwired: 2 in, 2 out]
              }
            }
          }
        }
        n247 = local read "STOP"() -> (w286:bool)
      }
      n248 = while {
        tunnel: refnum<visa-resource-name> "Lambda" ("VISA name") -> [w245]
        stop <- w244 stop-if-true
        # "Aquisição - Fonte DC"
        n249 = call <instrlib>:"GENie Meas Output Voltage.vi"("VISA"=w245) -> ("Output Voltage"=→"Tensão de saída":dbl, "VISA out"=w248:refnum<visa-resource-name>)  [unwired: 8 in, 1 out]
        n250 = Wait (ms)(milliseconds to wait=u32 200) -> ()  [unwired: 1 out]
        n251 = call <instrlib>:"GENie Meas Output Current.vi"("VISA"=w248) -> ("Output Current"=→"Corrente de saída":dbl)  [unwired: 8 in, 2 out]
        n252 = local read "STOP"() -> (w244:bool)
      }
      n253 = while {
        tunnel: w41 -> [w193]
        stop <- w179 stop-if-true
        # "Termopar Dissipador"
        # "Termopar uC IC601"
        # "Termopar Cap 504"
        # "Termopar Cap C112"
        # "Termopar Indutor L100"
        # "Termopar  IC100"
        # "Termopar Conector"
        # "Termopar Fusivel"
        # "Termopar Cap C006"
        # "tempo(s):"
        # "Termopar Cap C011"
        # "Termopar Cap C009"
        # "Termopar Choke L001"
        # "Gerando log das Temperaturas dos Termopares"
        n254 = local read "TP 3"() -> (w189:dbl)
        n255 = local read "TP 5"() -> (w176:dbl)
        n256 = local read "TP 6"() -> (w175:dbl)
        n257 = local read "TP 7"() -> (w172:dbl)
        n258 = local read "TP 8"() -> (w171:dbl)
        n259 = local read "TP 10"() -> (w168:dbl)
        n260 = local read "TP 11"() -> (w167:dbl)
        n261 = local read "TP 12"() -> (w164:dbl)
        n262 = local read "TP 15"() -> (w161:dbl)
        n263 = Wait (ms)(milliseconds to wait=u32 1000) -> ()  [unwired: 1 out]
        n264 = local read "TP 1"() -> (w178:dbl)
        n265 = local read "TP 2"() -> (w183:dbl)
        n266 = local read "Time"() -> (w187:dbl)
        n267 = local read "TP 13"() -> (w163:dbl)
        n268 = Number To Fractional String(number=w187, precision (6)=i16 3) -> (F-format string=w186:string)  [unwired: 2 in]
        n269 = Number To Fractional String(number=w178, precision (6)=i16 3) -> (F-format string=w185:string)  [unwired: 2 in]
        n270 = Number To Fractional String(number=w183, precision (6)=i16 3) -> (F-format string=w181:string)  [unwired: 2 in]
        n271 = Number To Exponential String(number=w189, precision (6)=i16 3) -> (E-format string=w191:string)  [unwired: 2 in]
        n272 = Number To Exponential String(number=w176, precision (6)=i16 3) -> (E-format string=w160:string)  [unwired: 2 in]
        n273 = Number To Exponential String(number=w175, precision (6)=i16 3) -> (E-format string=w159:string)  [unwired: 2 in]
        n274 = Number To Exponential String(number=w172, precision (6)=i16 3) -> (E-format string=w158:string)  [unwired: 2 in]
        n275 = Number To Exponential String(number=w171, precision (6)=i16 3) -> (E-format string=w157:string)  [unwired: 2 in]
        n276 = Number To Exponential String(number=w168, precision (6)=i16 3) -> (E-format string=w156:string)  [unwired: 2 in]
        n277 = Number To Exponential String(number=w167, precision (6)=i16 3) -> (E-format string=w155:string)  [unwired: 2 in]
        n278 = Number To Exponential String(number=w164, precision (6)=i16 3) -> (E-format string=w154:string)  [unwired: 2 in]
        n279 = Number To Exponential String(number=w163, precision (6)=i16 3) -> (E-format string=w153:string)  [unwired: 2 in]
        n280 = Number To Exponential String(number=w161, precision (6)=i16 3) -> (E-format string=w152:string)  [unwired: 2 in]
        n281 = Build Array(w186, w185, w181, w191, w160, w159, w158, w157, w156, w155, w154, w153, w152) -> (w182:string[])
        n282 = local read "STOP"() -> (w179:bool)
        n283 = call-poly <vilib>:"Write Delimited Spreadsheet.vi"("file path (dialog if empty)"=w193, "1D data"=w182, "append to file? (new file:F)"=TRUE, "transpose? (no:F)"=FALSE) -> ()  [unwired: 10 in, 2 out]
      }
    }
    frame #2 {
      n284 = local write "STOP"(FALSE ("STOP")) -> ()
    }
  }
